vi "ReportADCResultsinVoltsBB.vi"(8 "error in (no error)":errorcluster, 10 "Message IN":string, 11 "Blue Board Enum":T1) -> (0 "error out":errorcluster, 1 "Result":dbl, 2 "Message Out":string, 3 "VISA resource name out":refnum<visa-resource-name>)   [LabVIEW 2022 SP3]
uses:
  ADCSelector BB.ctl
  <vilib>/Instr/_visa.llb/VISA Flush IO Buffer Mask.ctl
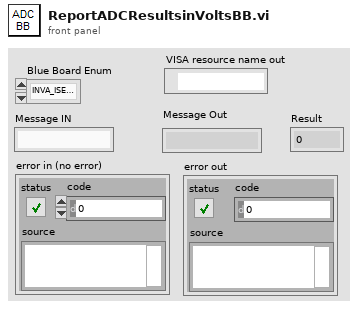
[diagram p1: front panel]
types:
  T1 = typedef "ADCSelector BB.ctl" = enum16{"INVA_ISENSE_U", "INVA_ISENSE_V", "INVA_ISENSE_W", "INVA_UDC", "INVA_TEMP", "HB_TEMP", "AUXB_TEMP", "VLINE_AB", "VLINE_BC", "VLINE_CA", "VSENSE_POS_24V", "VSENSE_POS_5V", "VSENSE_NEG_15V", "INVB_ISENSE_U", "INV_B_ISENSEV", "INVB_ISENSE_W", "INVB_UDC", "INVB_TEMP", "AUXA_TEMP", "AUXC_TEMP", "VOUT_AB", "VOUT_BC", "VOUT_CA", "VSENSE_POS_15V", "VSENSE_POS_3P3V", "TEST_POINT"}
  T2 = typedef "VISA Flush IO Buffer Mask.ctl" = u16
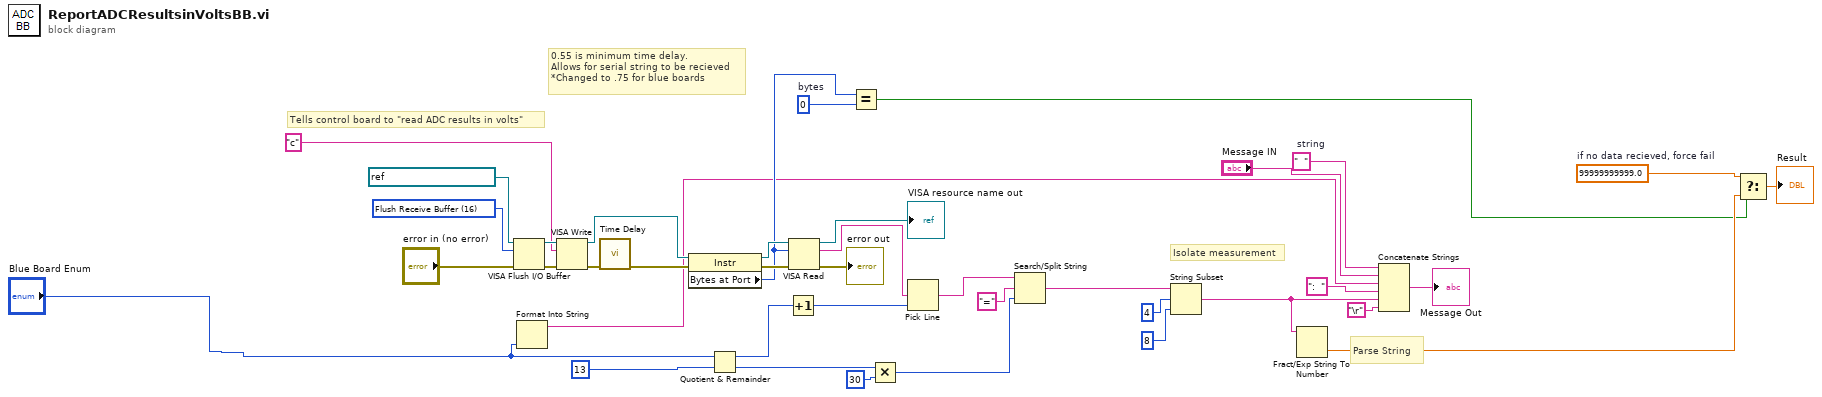
[diagram p0: block diagram]
diagram:
  w10 = "  "  # string
  w15 = 99999999999.0  # if no data recieved, force fail
  w18 = u32 0  # bytes
  w23 = T2 16 items=["Flush Receive Buffer"=16, "Write Transmit Buffer to Device"=32, "Flush Receive Buffer (No I/O)"=64, "Flush Transmit Buffer"=128] ("Mask")
  # "Isolate measurement"
  # "Parse String"
  # "0.55 is minimum time delay.\nAllows for serial string to be recieved\n*Changed to .75 for blue boards"
  # "Tells control board to \"read ADC results in volts\""
  n1 = VISA Flush I/O Buffer(VISA resource name=refnum<visa-resource-name> "ControlBoard", mask (16)=w23, error in (no error)="error in (no error)") -> (VISA resource name out=w25:refnum<visa-resource-name>, error out=w26:errorcluster)
  n2 = Format Into String("Blue Board Enum") -> (resulting string=w3:string)  [unwired: 3 in, 1 out]
  n3 = VISA Write(VISA resource name=w25, write buffer="c", error in (no error)=w26) -> (VISA resource name out=w28:refnum<visa-resource-name>, error out=w24:errorcluster)  [unwired: 1 out]
  n4 = call "Time Delay"("error in (no error)"=w24) -> ("error out"=w27:errorcluster)  [unwired: 10 in]
  n5 = property class="Instr"(reference=w28, error in=w27) -> (reference out=w21:refnum<visa-resource-name>, error out=w22:errorcluster, "Bytes at Port"=w19:u32)
  n6 = Quotient & Remainder(x="Blue Board Enum", y=13) -> (x-y*floor(x/y)=w32:i32, floor(x/y)=w34:i32)
  n7 = Increment(x=w32) -> (x+1=w33:i32)
  n8 = VISA Read(VISA resource name=w21, byte count=w19, error in (no error)=w22) -> (VISA resource name out=→"VISA resource name out":refnum<visa-resource-name>, read buffer=w37:string, error out=→"error out":errorcluster)  [unwired: 1 out]
  n9 = Equal?(x=w19, y=w18) -> (x = y?=w16:bool)
  n10 = Multiply(x=w34, y=30) -> (x*y=w36:i32)
  n11 = Pick Line(multi-line string=w37, line index=w33) -> (output string=w38:string)  [unwired: 1 in]
  n12 = Search/Split String(string=w38, search string/char (-)="=" ("regular expression"), offset (0)=w36) -> (match + rest of string=w30:string)  [unwired: 2 out]
  n13 = String Subset(string=w30, offset (0)=4, length (rest)=8 ("offset (0)")) -> (substring=w12:string)
  n14 = Fract/Exp String To Number(string=w12) -> (number=w17:dbl)  [unwired: 3 in, 1 out]
  n15 = Concatenate Strings(w10, "Message IN", w3, ":  ", w12, "\r") -> (→"Message Out":string)
  n16 = Select(t=w15, s=w16, f=w17) -> (s? t:f=→"Result":dbl)
